vi "Get IMAQdx Devices.vi"(8 "error in (no error)":errorcluster, 11 "Chosen Interface":string) -> (0 "error out":errorcluster, 1 "Interface Names":string[](array[string]), 2 "Row of Chosen Interface":i32, 3 "IMAQdx Devices":string[][](array[string]))   [LabVIEW 2012, in "Image UDP Broadcast Custom Device.lvlib"]
uses:
  Shared/Image UDP Broadcast Custom Device.lvlib
  <vilib>/vision/driver/NI_Vision_Acquisition_Software.lvlib
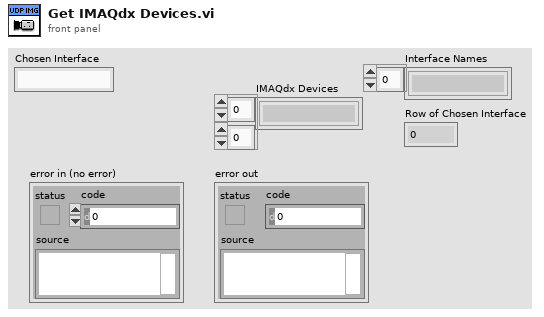
[diagram p1: front panel]
types:
  T1 = cluster{"Type":u32, "Version":u32, "Flags":u32, "SerialNumberHigh":u32, "SerialNumberLow":u32, "BusType":u32, "InterfaceName":string, "VendorName":string, "ModelName":string, "CameraFileName":string, "CameraAttributeURL":string}[]
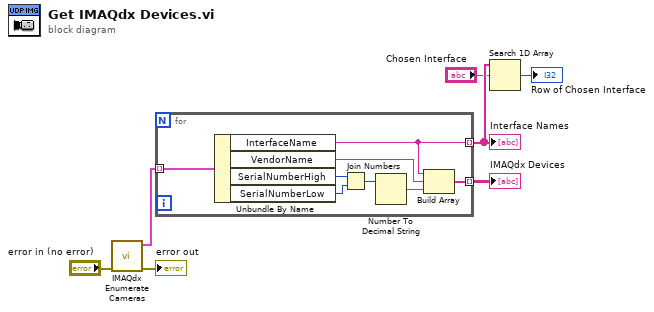
[diagram p0: block diagram]
diagram:
  n1 = call <vilib>:"IMAQdx Enumerate Cameras.vi"("error in"="error in (no error)") -> ("error out"=→"error out":errorcluster, "Camera Information Array"=w5:T1)  [unwired: 9 in]
  n2 = for {
    tunnel: w5 -> [w15] mode=indexing
    tunnel: [w12] -> w6 mode=indexing
    tunnel: [w8] -> w3 mode=indexing
    n3 = Unbundle By Name(w15) -> ("InterfaceName"=w8:string, "VendorName"=w9:string, "SerialNumberHigh"=w10:u32, "SerialNumberLow"=w14:u32)
    n4 = Join Numbers(hi=w10, lo=w14) -> ((hi.lo)=w13:u64)
    n5 = Number To Decimal String(number=w13) -> (decimal integer string=w11:string)  [unwired: 1 in]
    n6 = Build Array(w8, w9, w11) -> (w12:string[])
  }
  "IMAQdx Devices" <- w6
  "Interface Names" <- w3
  n7 = Search 1D Array(1D array=w3, element="Chosen Interface") -> (index of element=→"Row of Chosen Interface":i32)  [unwired: 1 in]
